vi "MOCK_FP_Read_Boolean.vi"(8 "error in (no error)":errorcluster, 11 "FieldPoint IO Point In":refnum<k21>) -> (0 "error out":errorcluster, 1 "timestamp":dbl format="%.2f", 2 "Boolean":bool=TRUE, 3 "FieldPoint IO Point Out":refnum<k21>)   [LabVIEW 2015]
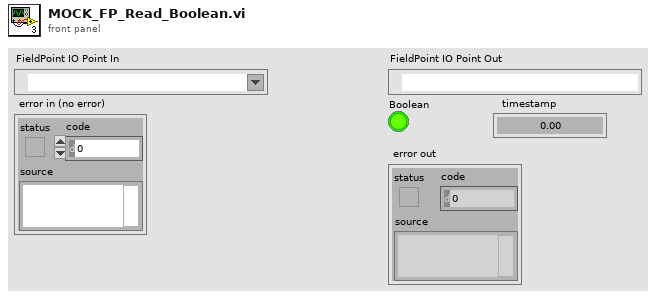
[diagram p1: front panel]
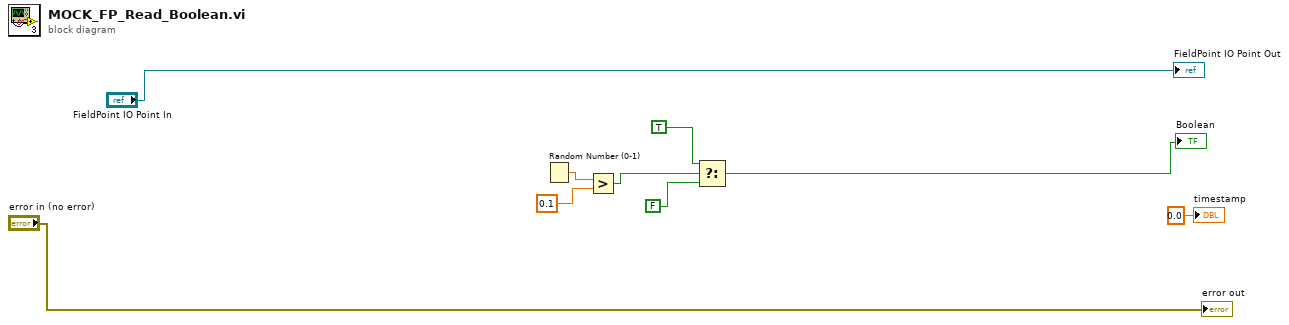
[diagram p0: block diagram]
diagram:
  n1 = Random Number (0-1)() -> (number: 0 to 1=w6:dbl)
  n2 = Greater?(x=w6, y=0.1) -> (0:w4:bool)
  n3 = Select(t=TRUE, s=w4, f=FALSE) -> (s? t:f=→"Boolean":bool)
  "FieldPoint IO Point Out" <- "FieldPoint IO Point In"
  "timestamp" <- 0.0 ("timestamp")
  "error out" <- "error in (no error)"
